vi "AutoUpdate.vi"(8 "error in (no error)":errorcluster, 10 "Node":refnum<k24>, 11 "List in":T1) -> (0 "error out":errorcluster, 3 "List out":T1)   [LabVIEW 2015, in "Workspace.Obejct.Radio.lvlib"]
uses:
  Workspace.Obejct.Radio.lvlib
  Types/Config.ctl
  NationalInstruments.VeriStand.SystemStorage
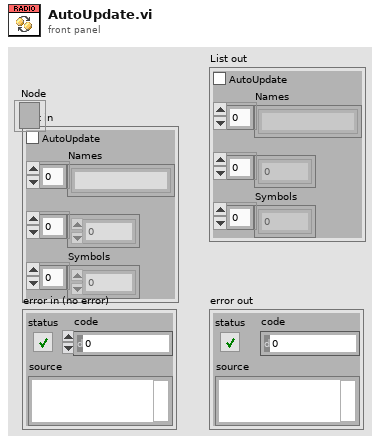
[diagram p1: front panel]
types:
  T1 = typedef "Workspace.Obejct.Radio.lvlib/Config.ctl" = cluster{"AutoUpdate":bool, "Names":string[], "Values":dbl[], "Symbols":i32[]}
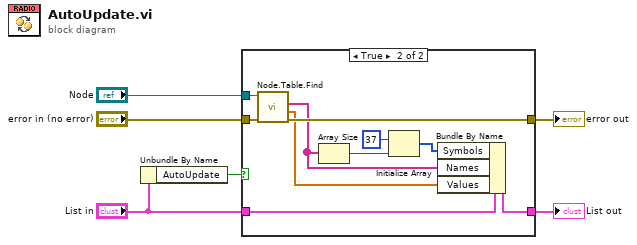
[diagram p0: block diagram]
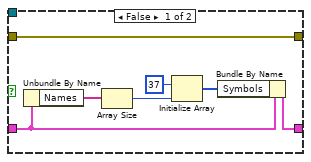
[diagram p2: hidden frame]
diagram:
  n1 = Unbundle By Name("List in") -> ("AutoUpdate"=w1:bool)
  n2 = case shown="True" w1 {
    tunnel: [w9 w23] -> w6
    tunnel: "List in" -> [w8 w22]
    tunnel: [w13 w21] -> w4
    tunnel: "error in (no error)" -> [w13 w20]
    tunnel: "Node" -> [_ w19]
    frame False {
      n3 = Unbundle By Name(w8) -> ("Names"=w7:string[])
      n4 = Array Size(array=w7) -> (size(s)=w12:i32)
      n5 = Initialize Array(37 ("element"), w12) -> (w10:i32[])
      n6 = Bundle By Name(cluster=w8, "Symbols"=w10) -> (w9:T1)
    }
    frame True {
      n7 = call "Node.Table.Find.vi"("error in (no error)"=w20, "Node"=w19) -> ("error out"=w21:errorcluster, "Values"=w18:dbl[], "Names"=w15:string[])  [unwired: 5 in, 2 out]
      n8 = Array Size(array=w15) -> (size(s)=w17:i32)
      n9 = Initialize Array(37 ("element"), w17) -> (w14:i32[])
      n10 = Bundle By Name(cluster=w22, "Symbols"=w14, "Names"=w15, "Values"=w18) -> (w23:T1)
    }
  }
  "List out" <- w6
  "error out" <- w4
